vi "Add Environment Devices.vi"(8 "Error In":errorcluster, 11 "IP Connection":refnum<class "IP Connection.lvclass">) -> (0 "Error Out":errorcluster, 1 "Humidity Bricklet":refnum<class "Humidity Bricklet.lvclass">, 2 "Temperature IR Bricklet":refnum<class "Temperature IR Bricklet.lvclass">, 3 "All Devices added?":bool, 4 "Ambient Light Bricklet":refnum<class "Ambient Light Bricklet.lvclass">, 6 "Barometer Bricklet":refnum<class "Barometer Bricklet.lvclass">)   [LabVIEW 2011]
doc: "This VI adds all bricklets necessary for a environmental datalogger or weather station. It adds a Temperature-IR, Humidity, Ambient Light and Barometer Bricklet."
uses:
  Classes/IP Connection/IP Connection.lvclass
  Classes/Ambient Light Bricklet/Ambient Light Bricklet.lvclass
  Classes/Barometer Bricklet/Barometer Bricklet.lvclass
  Classes/Humidity Bricklet/Humidity Bricklet.lvclass
  Classes/Temperature IR Bricklet/Temperature IR Bricklet.lvclass
  Classes/IP Connection/Properties/Read Enumerate Callback.vi
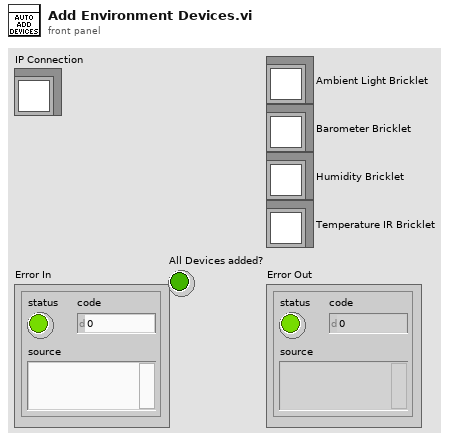
[diagram p1: front panel]
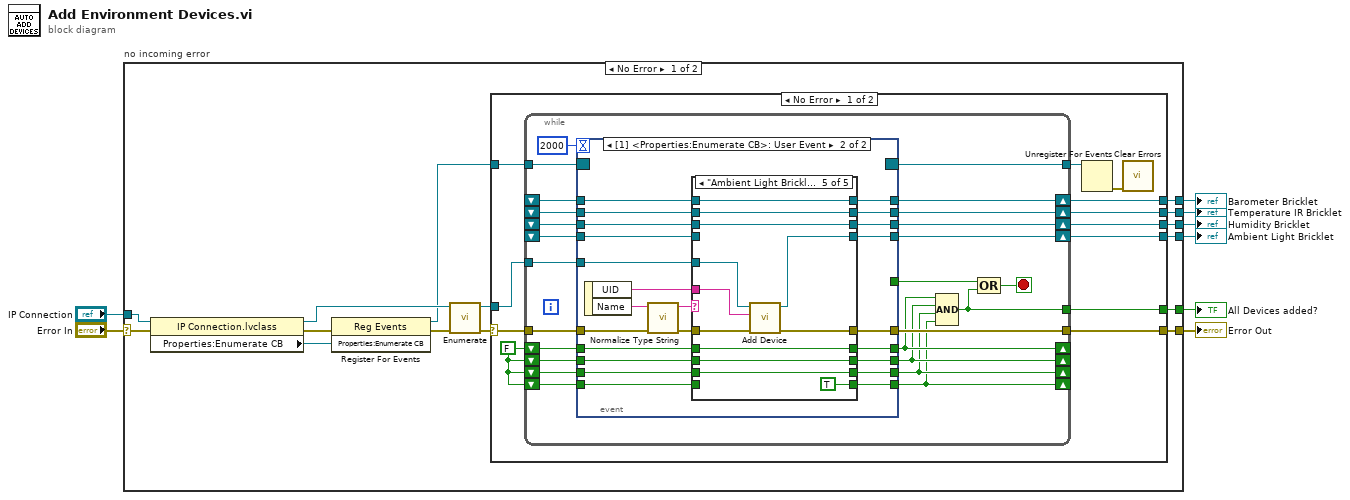
[diagram p0: block diagram]
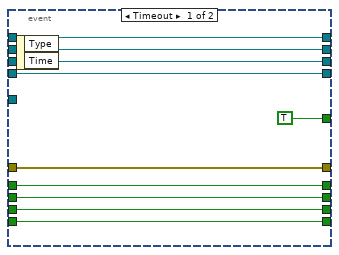
[diagram p2: hidden frame]
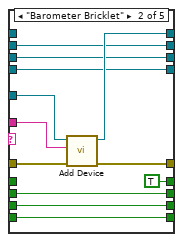
[diagram p4: hidden frame]
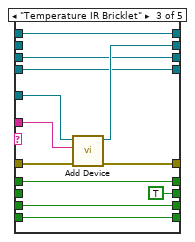
[diagram p5: hidden frame]
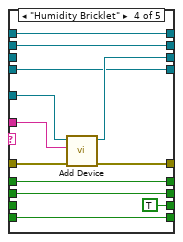
[diagram p6: hidden frame]
diagram:
  n1 = case "no incoming error" shown="No Error" "Error In" {
    selector: "Error In" -> [w23 w152]
    tunnel: [w14 w152] -> w7
    tunnel: "IP Connection" -> [w22 _]
    tunnel: [w13 _] -> w5
    tunnel: [w10 _] -> w4
    tunnel: [w9 _] -> w3
    tunnel: [w12 _] -> w2
    tunnel: [w11 _] -> w1
    frame No Error {
      n2 = property class="IP Connection.lvclass"(reference=w22, error in=w23) -> (reference out=w18:refnum<class "IP Connection.lvclass">, error out=w21:errorcluster, "Properties:Enumerate CB"=w20:refnum<user-event>)
      n3 = register-events(error in=w21, w20) -> (reference out=w16:refnum<event-registration>, error out=w19:errorcluster)  [unwired: 1 in]
      n4 = call "Enumerate.vi"("error in (no error)"=w19, "IP Connection in"=w18) -> ("error out"=w17:errorcluster, "IP Connection out"=w15:refnum<class "IP Connection.lvclass">)  [unwired: 8 in]
      n5 = case shown="No Error" w17 {
        selector: w17 -> [w34 w151]
        tunnel: w16 -> [w35 _]
        tunnel: w15 -> [w33 _]
        tunnel: [w32 w151] -> w14
        tunnel: [w29 _] -> w13
        tunnel: [w27 _] -> w10
        tunnel: [w26 _] -> w9
        tunnel: [w25 _] -> w12
        tunnel: [w24 _] -> w11
        frame No Error {
          w31 = FALSE
          n6 = while {
            tunnel: w35 -> [w60]
            tunnel: w34 -> [w59]
            tunnel: w33 -> [w58]
            tunnel: [w57] -> w32
            shift-right: [w56] -> w27
            shift-left: _ -> [w55]
            shift-right: [w54] -> w26
            shift-left: _ -> [w53]
            shift-right: [w52] -> w25
            shift-left: _ -> [w51]
            shift-right: [w50] -> w24
            shift-left: _ -> [w49]
            shift-right: [w43] -> _
            shift-left: w31 -> [w47]
            shift-right: [w42] -> _
            shift-left: w31 -> [w46]
            shift-right: [w41] -> _
            shift-left: w31 -> [w45]
            shift-right: [w40] -> _
            shift-left: w31 -> [w44]
            tunnel: [w37] -> w30
            tunnel: [w36] -> w29
            stop <- w39 stop-if-true
            n7 = event shown="[1] <Properties:Enumerate CB>: User Event" {
              selector: w60 -> [_ _]
              dyn-events: [_ _] -> w37
              timeout: 2000 -> [_ _]
              tunnel: w59 -> [w61 w93]
              tunnel: w58 -> [_ w88]
              tunnel: [w61 w87] -> w57
              tunnel: [w70 w86] -> w56
              tunnel: w55 -> [w70 w85]
              tunnel: [w69 w84] -> w54
              tunnel: w53 -> [w69 w83]
              tunnel: [w68 w82] -> w52
              tunnel: w51 -> [w68 w81]
              tunnel: [w67 w80] -> w50
              tunnel: w49 -> [w67 w79]
              tunnel: [w66 w78] -> w43
              tunnel: w47 -> [w66 w77]
              tunnel: [w65 w76] -> w42
              tunnel: w46 -> [w65 w75]
              tunnel: [w64 w74] -> w41
              tunnel: w45 -> [w64 w73]
              tunnel: [w63 w72] -> w40
              tunnel: w44 -> [w63 w71]
              tunnel: [TRUE _] -> w38
              event Timeout {
                n8 = event-data() -> ()  [unwired: 1 in, 2 out]
              }
              event User Event {
                n9 = event-data() -> ("UID"=w89:string, "Name"=w91:string)  [unwired: 1 in]
                n10 = call "Normalize Type String.vi"("Error In"=w93, "Name"=w91) -> ("Error Out"=w92:errorcluster, "normalized Name"=w90:string)  [unwired: 8 in]
                n11 = case shown="\"Ambient Light Bricklet\"" w90 {
                  tunnel: w92 -> [w101 w114 w126 w136 w148]
                  tunnel: w89 -> [_ w113 w125 w137 w149]
                  tunnel: w88 -> [_ w112 w124 w138 w150]
                  tunnel: [w101 w111 w123 w135 w147] -> w87
                  tunnel: [w102 w110 w119 w132 w143] -> w86
                  tunnel: w85 -> [w102 _ w119 w132 w143]
                  tunnel: [w100 w109 w122 w134 w146] -> w84
                  tunnel: w83 -> [w100 w109 _ w134 w146]
                  tunnel: [w99 w108 w121 w133 w145] -> w82
                  tunnel: w81 -> [w99 w108 w121 _ w145]
                  tunnel: [w98 w107 w120 w131 w144] -> w80
                  tunnel: w79 -> [w98 w107 w120 w131 _]
                  tunnel: [w97 TRUE w118 w130 w142] -> w78
                  tunnel: w77 -> [w97 _ w118 w130 w142]
                  tunnel: [w96 w105 TRUE w129 w141] -> w76
                  tunnel: w75 -> [w96 w105 _ w129 w141]
                  tunnel: [w95 w104 w116 TRUE w140] -> w74
                  tunnel: w73 -> [w95 w104 w116 _ w140]
                  tunnel: [w94 w103 w115 w127 TRUE] -> w72
                  tunnel: w71 -> [w94 w103 w115 w127 _]
                  frame Default {
                  }
                  frame "Barometer Bricklet" {
                    n12 = call "Add Device.vi"("Error In"=w114, "Device UID"=w113, "IP Connection"=w112) -> ("Error Out"=w111:errorcluster, "Barometer Bricklet"=w110:refnum<class "Barometer Bricklet.lvclass">)  [unwired: 7 in]
                  }
                  frame "Temperature IR Bricklet" {
                    n13 = call "Add Device.vi"("Error In"=w126, "Device UID"=w125, "IP Connection"=w124) -> ("Error Out"=w123:errorcluster, "Ambient Light Bricklet"=w122:refnum<class "Temperature IR Bricklet.lvclass">)  [unwired: 7 in]
                  }
                  frame "Humidity Bricklet" {
                    n14 = call "Add Device.vi"("Error In"=w136, "Device UID"=w137, "IP Connection"=w138) -> ("Error Out"=w135:errorcluster, "Humidity Bricklet"=w133:refnum<class "Humidity Bricklet.lvclass">)  [unwired: 7 in]
                  }
                  frame "Ambient Light Bricklet" {
                    n15 = call "Add Device.vi"("Error In"=w148, "Device UID"=w149, "IP Connection"=w150) -> ("Error Out"=w147:errorcluster, "Ambient Light Bricklet"=w144:refnum<class "Ambient Light Bricklet.lvclass">)  [unwired: 7 in]
                  }
                }
              }
            }
            n16 = Compound Arithmetic op=AND(w43, w42, w41, w40) -> (w36:bool)
            n17 = Compound Arithmetic op=OR(w38, w36) -> (w39:bool)
          }
          n18 = Unregister For Events(event registration refnum=w30) -> (error out=w28:errorcluster)  [unwired: 1 in]
          n19 = call <vilib>:"Clear Errors.vi"("error in (no error)"=w28) -> ()  [unwired: 6 in, 1 out]
        }
        frame Error {
        }
      }
    }
    frame Error {
    }
  }
  "Error Out" <- w7
  "Ambient Light Bricklet" <- w1
  "Barometer Bricklet" <- w4
  "All Devices added?" <- w5
  "Humidity Bricklet" <- w2
  "Temperature IR Bricklet" <- w3
